vi "输入数据解析.vi"(0 "单个参数补充":dbl, 1 "从板号":dbl=1.0, 2 "主板二维码":string="BNET01", 3 "从板二维码":string="BNET01", 5 "主板引用":refnum<vi>, 7 "从板引用":refnum<vi>, 9 "主板选项":string="三级故障阀值", 11 "枚举":enum16{"主板", "从板"}(ring), 12 "快换":bool caption="快换写入") -> (4 "输出数组":dbl[][](array[numeric]), 6 "数组长度":dbl[](array[numeric]), 8 "循环次数":i32, 10 "命令":u32, 14 "名称":string[](array[string]), 15 "命令序号":u32[](array[numeric]))   [LabVIEW 2013] (continued)
                    n998 = Unbundle By Name(w2451) -> ("整组温度不均衡"=w2450:dbl)
                    n999 = call "输入分辨率计算-EV05.vi"("1字节?"=TRUE, "数值"=w2450, "偏移量"=0.0, "分辨率"=1.0) -> ("高字节1"=w2453:dbl)  [unwired: 1 in, 6 out]
                  }
                  frame Enabled {
                  }
                }
                n1000 = Build Array(w2449) -> (w2448:i32[])
              }
              frame 5 {
                # "单组电压不均衡"
                n1001 = disable-structure shown="启用" {
                  disable-tunnel: [w2465 w2468] -> w2460
                  disable-tunnel: [w2463 w2468] -> w2458
                  disable-tunnel: w2457 -> [w2462 _]
                  frame Disabled {
                    n1002 = Unbundle By Name(w2462) -> ("单组电压不均衡"=w2461:dbl)
                    n1003 = call "输入分辨率计算-EV05.vi"("1字节?"=FALSE, "数值"=w2461, "偏移量"=0.0, "分辨率"=0.001) -> ("低字节"=w2463:dbl, "高字节1"=w2465:dbl)  [unwired: 1 in, 5 out]
                  }
                  frame Enabled {
                    w2468 = 255 ("高字节1")
                  }
                }
                n1004 = Build Array(w2460, w2458) -> (w2459:i32[])
              }
              frame 6 {
                # "整组电压不均衡"
                n1005 = disable-structure shown="启用" {
                  disable-tunnel: [w2477 w2480] -> w2472
                  disable-tunnel: [w2475 w2480] -> w2470
                  disable-tunnel: w2469 -> [w2474 _]
                  frame Disabled {
                    n1006 = Unbundle By Name(w2474) -> ("整组电压不均衡"=w2473:dbl)
                    n1007 = call "输入分辨率计算-EV05.vi"("1字节?"=FALSE, "数值"=w2473, "偏移量"=0.0, "分辨率"=0.001) -> ("低字节"=w2475:dbl, "高字节1"=w2477:dbl)  [unwired: 1 in, 5 out]
                  }
                  frame Enabled {
                    w2480 = 255 ("高字节1")
                  }
                }
                n1008 = Build Array(w2472, w2470) -> (w2471:i32[])
              }
              frame 7 {
                # "单体电压过高"
                n1009 = disable-structure shown="启用" {
                  disable-tunnel: [w2489 w2492] -> w2484
                  disable-tunnel: [w2487 w2492] -> w2482
                  disable-tunnel: w2481 -> [w2486 _]
                  frame Disabled {
                    n1010 = Unbundle By Name(w2486) -> ("单体电压过高"=w2485:dbl)
                    n1011 = call "输入分辨率计算-EV05.vi"("1字节?"=FALSE, "数值"=w2485, "偏移量"=0.0, "分辨率"=0.001) -> ("低字节"=w2487:dbl, "高字节1"=w2489:dbl)  [unwired: 1 in, 5 out]
                  }
                  frame Enabled {
                    w2492 = 255 ("高字节1")
                  }
                }
                n1012 = Build Array(w2484, w2482) -> (w2483:i32[])
              }
              frame 8 {
                # "单体电压过低"
                n1013 = disable-structure shown="启用" {
                  disable-tunnel: [w2501 w2504] -> w2496
                  disable-tunnel: [w2499 w2504] -> w2494
                  disable-tunnel: w2493 -> [w2498 _]
                  frame Disabled {
                    n1014 = Unbundle By Name(w2498) -> ("单体电压过低"=w2497:dbl)
                    n1015 = call "输入分辨率计算-EV05.vi"("1字节?"=FALSE, "数值"=w2497, "偏移量"=0.0, "分辨率"=0.001) -> ("低字节"=w2499:dbl, "高字节1"=w2501:dbl)  [unwired: 1 in, 5 out]
                  }
                  frame Enabled {
                    w2504 = 255 ("高字节1")
                  }
                }
                n1016 = Build Array(w2496, w2494) -> (w2495:i32[])
              }
              frame 9 {
                # "充电电流过高"
                n1017 = disable-structure shown="启用" {
                  disable-tunnel: [w2513 w2516] -> w2508
                  disable-tunnel: [w2511 w2516] -> w2506
                  disable-tunnel: w2505 -> [w2510 _]
                  frame Disabled {
                    n1018 = Unbundle By Name(w2510) -> ("充电电流过高"=w2509:dbl)
                    n1019 = call "输入分辨率计算-EV05.vi"("1字节?"=FALSE, "数值"=w2509, "偏移量"=-3000.0, "分辨率"=0.1) -> ("低字节"=w2511:dbl, "高字节1"=w2513:dbl)  [unwired: 1 in, 5 out]
                  }
                  frame Enabled {
                    w2516 = 255 ("高字节1")
                  }
                }
                n1020 = Build Array(w2508, w2506) -> (w2507:i32[])
              }
              frame 10 {
                # "放电电流过高"
                n1021 = disable-structure shown="启用" {
                  disable-tunnel: [w2525 w2528] -> w2520
                  disable-tunnel: [w2523 w2528] -> w2518
                  disable-tunnel: w2517 -> [w2522 _]
                  frame Disabled {
                    n1022 = Unbundle By Name(w2522) -> ("放电电流过高"=w2521:dbl)
                    n1023 = call "输入分辨率计算-EV05.vi"("1字节?"=FALSE, "数值"=w2521, "偏移量"=-3000.0, "分辨率"=0.1) -> ("低字节"=w2523:dbl, "高字节1"=w2525:dbl)  [unwired: 1 in, 5 out]
                  }
                  frame Enabled {
                    w2528 = 255 ("高字节1")
                  }
                }
                n1024 = Build Array(w2520, w2518) -> (w2519:i32[])
              }
              frame 11 {
                # "单组温度不均衡"
                n1025 = disable-structure shown="启用" {
                  disable-tunnel: [w2535 255 ("高字节1")] -> w2531
                  disable-tunnel: w2529 -> [w2533 _]
                  frame Disabled {
                    n1026 = Unbundle By Name(w2533) -> ("单组温度不均衡"=w2532:dbl)
                    n1027 = call "输入分辨率计算-EV05.vi"("1字节?"=TRUE, "数值"=w2532, "偏移量"=0.0, "分辨率"=1.0) -> ("高字节1"=w2535:dbl)  [unwired: 1 in, 6 out]
                  }
                  frame Enabled {
                  }
                }
                n1028 = Build Array(w2531) -> (w2530:i32[])
              }
              frame 12 {
                # "SOC过高"
                n1029 = Unbundle By Name(w2543) -> ("SOC过高"=w2542:dbl)
                n1030 = call "输入分辨率计算-EV05.vi"("1字节?"=FALSE, "数值"=w2542, "偏移量"=0.0, "分辨率"=0.1) -> ("低字节"=w2544:dbl, "高字节1"=w2545:dbl)  [unwired: 1 in, 5 out]
                n1031 = call "二进制解析-8.6.vi"("索引"=4, "数值"=w2545) -> ("低位子数组"=w2548:i32[])  [unwired: 3 out]
                n1032 = call "二进制解析-8.6.vi"("索引"=4, "数值"=w2544) -> ("低位子数组"=w2540:i32[], "高位子数组"=w2547:i32[])  [unwired: 2 out]
                n1033 = Insert Into Array(array=w2548, new element=w2547) -> (w2546:i32[])  [unwired: 1 in]
                n1034 = call "数值二进制转十进制-8.6.vi"("子数组"=w2546) -> ("十进制数值"=w2541:i32)  [unwired: 4 out]
                n1035 = disable-structure shown="启用" {
                  disable-tunnel: w2541 -> [w2556 _]
                  disable-tunnel: [w2556 255 ("高字节1")] -> w2539
                  disable-tunnel: [w2555 i32[] [] ("低位子数组 20")] -> _
                  disable-tunnel: w2540 -> [w2555 _]
                  frame Disabled {
                  }
                  frame Enabled {
                  }
                }
                n1036 = Build Array(w2539, w2539) -> (w2552:i32[])
              }
              frame 13 {
                # "SOC过低"
                n1037 = Unbundle By Name(w2565) -> ("SOC过低"=w2564:dbl)
                n1038 = call "输入分辨率计算-EV05.vi"("1字节?"=FALSE, "数值"=w2564, "偏移量"=0.0, "分辨率"=0.1) -> ("低字节"=w2562:dbl, "高字节1"=w2563:dbl)  [unwired: 1 in, 5 out]
                n1039 = call "二进制解析-8.6.vi"("索引"=4, "数值"=w2563) -> ("低位子数组"=w2560:i32[])  [unwired: 3 out]
                n1040 = disable-structure shown="启用" {
                  disable-tunnel: w2562 -> [w2572 _]
                  disable-tunnel: [w2572 255 ("高字节1")] -> w2561
                  disable-tunnel: w2560 -> [w2571 _]
                  disable-tunnel: [_ 255 ("高字节1")] -> w2559
                  frame Disabled {
                    (unwired) i32[] [] ("低位子数组 4")
                  }
                  frame Enabled {
                  }
                }
                n1041 = Build Array(w2559, w2561) -> (w2568:i32[])
              }
              frame 14 {
                # "内阻过大"
                n1042 = disable-structure shown="启用" {
                  disable-tunnel: w2577 -> [w2582 _]
                  disable-tunnel: [w2578 255 ("高字节1")] -> w2575
                  frame Disabled {
                    n1043 = Unbundle By Name(w2582) -> ("内阻过大"=w2581:dbl)
                    n1044 = call "输入分辨率计算-EV05.vi"("1字节?"=TRUE, "数值"=w2581, "分辨率"=0.1) -> ("高字节1"=w2578:dbl)  [unwired: 2 in, 6 out]
                  }
                  frame Enabled {
                  }
                }
                n1045 = Build Array(w2575) -> (w2576:i32[])
              }
              frame 15 {
                # "极柱温度过高"
                n1046 = disable-structure shown="启用" {
                  disable-tunnel: w2586 -> [w2592 _]
                  disable-tunnel: [w2588 255 ("高字节1")] -> w2584
                  frame Disabled {
                    n1047 = Unbundle By Name(w2592) -> ("极柱温度过高"=w2591:dbl)
                    n1048 = call "输入分辨率计算-EV05.vi"("1字节?"=TRUE, "数值"=w2591, "偏移量"=-40.0, "分辨率"=1.0) -> ("高字节1"=w2588:dbl)  [unwired: 1 in, 6 out]
                  }
                  frame Enabled {
                  }
                }
                n1049 = Build Array(w2584) -> (w2585:i32[])
              }
              frame 16 {
                # "SOH过低"
                n1050 = disable-structure shown="启用" {
                  disable-tunnel: [w2609 w2617] -> w2596
                  disable-tunnel: w2595 -> [w2606 _]
                  disable-tunnel: [w2598 w2617] -> w2594
                  frame Disabled {
                    n1051 = Unbundle By Name(w2606) -> ("SOH过低"=w2605:dbl)
                    n1052 = call "输入分辨率计算-EV05.vi"("1字节?"=FALSE, "数值"=w2605, "偏移量"=0.0, "分辨率"=0.1) -> ("低字节"=w2607:dbl, "高字节1"=w2608:dbl)  [unwired: 1 in, 5 out]
                    n1053 = call "二进制解析-8.6.vi"("索引"=4, "数值"=w2608) -> ("低位子数组"=w2611:i32[])  [unwired: 3 out]
                    n1054 = call "二进制解析-8.6.vi"("索引"=4, "数值"=w2607) -> ("低位子数组"=w2600:i32[], "高位子数组"=w2610:i32[])  [unwired: 2 out]
                    n1055 = call "二进制解析-8.6.vi"("索引"=4, "数值"=0) -> ("低位子数组"=w2601:i32[])  [unwired: 3 out]
                    n1056 = Insert Into Array(array=w2611, new element=w2610) -> (w2604:i32[])  [unwired: 1 in]
                    n1057 = Insert Into Array(array=w2600, new element=w2601) -> (w2599:i32[])  [unwired: 1 in]
                    n1058 = call "数值二进制转十进制-8.6.vi"("子数组"=w2604) -> ("十进制数值"=w2609:i32)  [unwired: 4 out]
                    n1059 = call "数值二进制转十进制-8.6.vi"("子数组"=w2599) -> ("十进制数值"=w2598:i32)  [unwired: 4 out]
                  }
                  frame Enabled {
                    w2617 = 255 ("高字节1")
                  }
                }
                n1060 = Build Array(w2596, w2594) -> (w2597:i32[])
              }
            }
            n1061 = Insert Into Array(array=w2401, new element=w2402) -> (w2400:dbl[])  [unwired: 1 in]
          }
          n1062 = Build Array(w2397) -> (w2396:dbl[][])
          n1063 = Build Array("三级故障阀值") -> (w2387:string[])
        }
        frame "温度过高(2)" {
          n1064 = Unbundle By Name(w2623) -> ("一级故障 2"=w2624:refnum<vi>)
          n1065 = property class="Clust (严格)"(reference=w2624) -> ("Value"=w2622:T4)  [unwired: 1 in, 2 out]
          n1066 = for {
            N: 17 -> [_]
            tunnel: w2622 -> [w2634]
            shift-right: [w2631] -> w2628
            shift-left: dbl[] [] -> [w2632]
            i -> [w2635]
            n1067 = case shown="13" w2635 {
              tunnel: w2634 -> [w2636 w2647 w2658 w2668 w2678 w2688 w2700 w2712 w2724 w2736 w2748 w2760 w2774 w2796 w2808 w2817 w2826]
              tunnel: [w2637 w2648 w2659 w2669 w2679 w2690 w2702 w2714 w2726 w2738 w2750 w2761 w2783 w2799 w2807 w2816 w2828] -> w2633
              frame 0, Default {
                # "总电压过高"
                n1068 = disable-structure shown="启用" {
                  disable-tunnel: [w2643 w2646] -> w2639
                  disable-tunnel: [w2642 w2646] -> w2638
                  disable-tunnel: w2636 -> [w2641 _]
                  frame Disabled {
                    n1069 = Unbundle By Name(w2641) -> ("总电压过高"=w2640:dbl)
                    n1070 = call "输入分辨率计算-EV05.vi"("1字节?"=FALSE, "数值"=w2640, "分辨率"=0.1) -> ("低字节"=w2643:dbl, "高字节1"=w2642:dbl)  [unwired: 2 in, 5 out]
                  }
                  frame Enabled {
                    w2646 = 255 ("高字节1")
                  }
                }
                n1071 = Build Array(w2638, w2639) -> (w2637:i32[])
              }
              frame 1 {
                # "总电压过低"
                n1072 = disable-structure shown="启用" {
                  disable-tunnel: [w2654 w2657] -> w2650
                  disable-tunnel: [w2653 w2657] -> w2649
                  disable-tunnel: w2647 -> [w2652 _]
                  frame Disabled {
                    n1073 = Unbundle By Name(w2652) -> ("总电压过低"=w2651:dbl)
                    n1074 = call "输入分辨率计算-EV05.vi"("1字节?"=FALSE, "数值"=w2651, "分辨率"=0.1) -> ("低字节"=w2654:dbl, "高字节1"=w2653:dbl)  [unwired: 2 in, 5 out]
                  }
                  frame Enabled {
                    w2657 = 255 ("高字节1")
                  }
                }
                n1075 = Build Array(w2649, w2650) -> (w2648:i32[])
              }
              frame 2 {
                # "温度过高"
                n1076 = disable-structure shown="启用" {
                  disable-tunnel: [w2664 255 ("高字节1")] -> w2660
                  disable-tunnel: w2658 -> [w2662 _]
                  frame Enabled {
                    n1077 = Unbundle By Name(w2662) -> ("温度过高"=w2661:dbl)
                    n1078 = call "输入分辨率计算-EV05.vi"("1字节?"=TRUE, "数值"=w2661, "偏移量"=-40.0, "分辨率"=1.0) -> ("高字节1"=w2664:dbl)  [unwired: 1 in, 6 out]
                  }
                  frame Disabled {
                  }
                }
                n1079 = Build Array(w2660) -> (w2659:dbl[])
              }
              frame 3 {
                # "温度过低"
                n1080 = disable-structure shown="启用" {
                  disable-tunnel: [w2674 255 ("高字节1")] -> w2670
                  disable-tunnel: w2668 -> [w2672 _]
                  frame Disabled {
                    n1081 = Unbundle By Name(w2672) -> ("温度过低"=w2671:dbl)
                    n1082 = call "输入分辨率计算-EV05.vi"("1字节?"=TRUE, "数值"=w2671, "偏移量"=-40.0, "分辨率"=1.0) -> ("高字节1"=w2674:dbl)  [unwired: 1 in, 6 out]
                  }
                  frame Enabled {
                  }
                }
                n1083 = Build Array(w2670) -> (w2669:i32[])
              }
              frame 4 {
                # "整组温度不均衡"
                n1084 = disable-structure shown="启用" {
                  disable-tunnel: [w2684 255 ("高字节1")] -> w2680
                  disable-tunnel: w2678 -> [w2682 _]
                  frame Disabled {
                    n1085 = Unbundle By Name(w2682) -> ("整组温度不均衡"=w2681:dbl)
                    n1086 = call "输入分辨率计算-EV05.vi"("1字节?"=TRUE, "数值"=w2681, "偏移量"=0.0, "分辨率"=1.0) -> ("高字节1"=w2684:dbl)  [unwired: 1 in, 6 out]
                  }
                  frame Enabled {
                  }
                }
                n1087 = Build Array(w2680) -> (w2679:i32[])
              }
              frame 5 {
                # "单组电压不均衡"
                n1088 = disable-structure shown="启用" {
                  disable-tunnel: [w2696 w2699] -> w2691
                  disable-tunnel: [w2694 w2699] -> w2689
                  disable-tunnel: w2688 -> [w2693 _]
                  frame Disabled {
                    n1089 = Unbundle By Name(w2693) -> ("单组电压不均衡"=w2692:dbl)
                    n1090 = call "输入分辨率计算-EV05.vi"("1字节?"=FALSE, "数值"=w2692, "偏移量"=0.0, "分辨率"=0.001) -> ("低字节"=w2694:dbl, "高字节1"=w2696:dbl)  [unwired: 1 in, 5 out]
                  }
                  frame Enabled {
                    w2699 = 255 ("高字节1")
                  }
                }
                n1091 = Build Array(w2691, w2689) -> (w2690:i32[])
              }
              frame 6 {
                # "整组电压不均衡"
                n1092 = disable-structure shown="启用" {
                  disable-tunnel: [w2708 w2711] -> w2703
                  disable-tunnel: [w2706 w2711] -> w2701
                  disable-tunnel: w2700 -> [w2705 _]
                  frame Disabled {
                    n1093 = Unbundle By Name(w2705) -> ("整组电压不均衡"=w2704:dbl)
                    n1094 = call "输入分辨率计算-EV05.vi"("1字节?"=FALSE, "数值"=w2704, "偏移量"=0.0, "分辨率"=0.001) -> ("低字节"=w2706:dbl, "高字节1"=w2708:dbl)  [unwired: 1 in, 5 out]
                  }
                  frame Enabled {
                    w2711 = 255 ("高字节1")
                  }
                }
                n1095 = Build Array(w2703, w2701) -> (w2702:i32[])
              }
              frame 7 {
                # "单体电压过高"
                n1096 = disable-structure shown="启用" {
                  disable-tunnel: [w2720 w2723] -> w2715
                  disable-tunnel: [w2718 w2723] -> w2713
                  disable-tunnel: w2712 -> [w2717 _]
                  frame Disabled {
                    n1097 = Unbundle By Name(w2717) -> ("单体电压过高"=w2716:dbl)
                    n1098 = call "输入分辨率计算-EV05.vi"("1字节?"=FALSE, "数值"=w2716, "偏移量"=0.0, "分辨率"=0.001) -> ("低字节"=w2718:dbl, "高字节1"=w2720:dbl)  [unwired: 1 in, 5 out]
                  }
                  frame Enabled {
                    w2723 = 255 ("高字节1")
                  }
                }
                n1099 = Build Array(w2715, w2713) -> (w2714:i32[])
              }
              frame 8 {
                # "单体电压过低"
                n1100 = disable-structure shown="启用" {
                  disable-tunnel: [w2732 w2735] -> w2727
                  disable-tunnel: [w2730 w2735] -> w2725
                  disable-tunnel: w2724 -> [w2729 _]
                  frame Disabled {
                    n1101 = Unbundle By Name(w2729) -> ("单体电压过低"=w2728:dbl)
                    n1102 = call "输入分辨率计算-EV05.vi"("1字节?"=FALSE, "数值"=w2728, "偏移量"=0.0, "分辨率"=0.001) -> ("低字节"=w2730:dbl, "高字节1"=w2732:dbl)  [unwired: 1 in, 5 out]
                  }
                  frame Enabled {
                    w2735 = 255 ("高字节1")
                  }
                }
                n1103 = Build Array(w2727, w2725) -> (w2726:i32[])
              }
              frame 9 {
                # "充电电流过高"
                n1104 = disable-structure shown="启用" {
                  disable-tunnel: [w2744 w2747] -> w2739
                  disable-tunnel: [w2742 w2747] -> w2737
                  disable-tunnel: w2736 -> [w2741 _]
                  frame Disabled {
                    n1105 = Unbundle By Name(w2741) -> ("充电电流过高"=w2740:dbl)
                    n1106 = call "输入分辨率计算-EV05.vi"("1字节?"=FALSE, "数值"=w2740, "偏移量"=-3000.0, "分辨率"=0.1) -> ("低字节"=w2742:dbl, "高字节1"=w2744:dbl)  [unwired: 1 in, 5 out]
                  }
                  frame Enabled {
                    w2747 = 255 ("高字节1")
                  }
                }
                n1107 = Build Array(w2739, w2737) -> (w2738:i32[])
              }
              frame 10 {
                # "放电电流过高"
                n1108 = disable-structure shown="启用" {
                  disable-tunnel: [w2756 w2759] -> w2751
                  disable-tunnel: [w2754 w2759] -> w2749
                  disable-tunnel: w2748 -> [w2753 _]
                  frame Disabled {
                    n1109 = Unbundle By Name(w2753) -> ("放电电流过高"=w2752:dbl)
                    n1110 = call "输入分辨率计算-EV05.vi"("1字节?"=FALSE, "数值"=w2752, "偏移量"=-3000.0, "分辨率"=0.1) -> ("低字节"=w2754:dbl, "高字节1"=w2756:dbl)  [unwired: 1 in, 5 out]
                  }
                  frame Enabled {
                    w2759 = 255 ("高字节1")
                  }
                }
                n1111 = Build Array(w2751, w2749) -> (w2750:i32[])
              }
              frame 11 {
                # "单组温度不均衡"
                n1112 = disable-structure shown="启用" {
                  disable-tunnel: [w2766 255 ("高字节1")] -> w2762
                  disable-tunnel: w2760 -> [w2764 _]
                  frame Disabled {
                    n1113 = Unbundle By Name(w2764) -> ("单组温度不均衡"=w2763:dbl)
                    n1114 = call "输入分辨率计算-EV05.vi"("1字节?"=TRUE, "数值"=w2763, "偏移量"=0.0, "分辨率"=1.0) -> ("高字节1"=w2766:dbl)  [unwired: 1 in, 6 out]
                  }
                  frame Enabled {
                  }
                }
                n1115 = Build Array(w2762) -> (w2761:i32[])
              }
              frame 12 {
                # "SOC过高"
                n1116 = Unbundle By Name(w2774) -> ("SOC过高"=w2773:dbl)
                n1117 = call "输入分辨率计算-EV05.vi"("1字节?"=FALSE, "数值"=w2773, "偏移量"=0.0, "分辨率"=0.1) -> ("低字节"=w2775:dbl, "高字节1"=w2776:dbl)  [unwired: 1 in, 5 out]
                n1118 = call "二进制解析-8.6.vi"("索引"=4, "数值"=w2776) -> ("低位子数组"=w2779:i32[])  [unwired: 3 out]
                n1119 = call "二进制解析-8.6.vi"("索引"=4, "数值"=w2775) -> ("低位子数组"=w2771:i32[], "高位子数组"=w2778:i32[])  [unwired: 2 out]
                n1120 = Insert Into Array(array=w2779, new element=w2778) -> (w2777:i32[])  [unwired: 1 in]
                n1121 = call "数值二进制转十进制-8.6.vi"("子数组"=w2777) -> ("十进制数值"=w2772:i32)  [unwired: 4 out]
                n1122 = disable-structure shown="启用" {
                  disable-tunnel: w2772 -> [w2787 _]
                  disable-tunnel: [w2787 255 ("高字节1")] -> w2770
                  disable-tunnel: [w2786 i32[] [] ("低位子数组 20")] -> _
                  disable-tunnel: w2771 -> [w2786 _]
                  frame Disabled {
                  }
                  frame Enabled {
                  }
                }
                n1123 = Build Array(w2770, w2770) -> (w2783:i32[])
              }
              frame 13 {
                # "SOC过低"
                n1124 = Unbundle By Name(w2796) -> ("SOC过低"=w2795:dbl)
                n1125 = call "输入分辨率计算-EV05.vi"("1字节?"=FALSE, "数值"=w2795, "偏移量"=0.0, "分辨率"=0.1) -> ("低字节"=w2793:dbl, "高字节1"=w2794:dbl)  [unwired: 1 in, 5 out]
                n1126 = call "二进制解析-8.6.vi"("索引"=4, "数值"=w2794) -> ("低位子数组"=w2791:i32[])  [unwired: 3 out]
                n1127 = disable-structure shown="启用" {
                  disable-tunnel: w2793 -> [w2803 _]
                  disable-tunnel: [w2803 255 ("高字节1")] -> w2792
                  disable-tunnel: w2791 -> [w2802 _]
                  disable-tunnel: [_ 255 ("高字节1")] -> w2790
                  frame Disabled {
                    (unwired) i32[] [] ("低位子数组 4")
                  }
                  frame Enabled {
                  }
                }
                n1128 = Build Array(w2790, w2792) -> (w2799:i32[])
              }
              frame 14 {
                # "内阻过大"
                n1129 = disable-structure shown="启用" {
                  disable-tunnel: w2808 -> [w2813 _]
                  disable-tunnel: [w2809 255 ("高字节1")] -> w2806
                  frame Disabled {
                    n1130 = Unbundle By Name(w2813) -> ("内阻过大"=w2812:dbl)
                    n1131 = call "输入分辨率计算-EV05.vi"("1字节?"=TRUE, "数值"=w2812, "分辨率"=0.1) -> ("高字节1"=w2809:dbl)  [unwired: 2 in, 6 out]
                  }
                  frame Enabled {
                  }
                }
                n1132 = Build Array(w2806) -> (w2807:i32[])
              }
              frame 15 {
                # "极柱温度过高"
                n1133 = disable-structure shown="启用" {
                  disable-tunnel: w2817 -> [w2823 _]
                  disable-tunnel: [w2819 255 ("高字节1")] -> w2815
                  frame Disabled {
                    n1134 = Unbundle By Name(w2823) -> ("极柱温度过高"=w2822:dbl)
                    n1135 = call "输入分辨率计算-EV05.vi"("1字节?"=TRUE, "数值"=w2822, "偏移量"=-40.0, "分辨率"=1.0) -> ("高字节1"=w2819:dbl)  [unwired: 1 in, 6 out]
                  }
                  frame Enabled {
                  }
                }
                n1136 = Build Array(w2815) -> (w2816:i32[])
              }
              frame 16 {
                # "SOH过低"
                n1137 = disable-structure shown="启用" {
                  disable-tunnel: [w2840 w2848] -> w2827
                  disable-tunnel: w2826 -> [w2837 _]
                  disable-tunnel: [w2829 w2848] -> w2825
                  frame Disabled {
                    n1138 = Unbundle By Name(w2837) -> ("SOH过低"=w2836:dbl)
                    n1139 = call "输入分辨率计算-EV05.vi"("1字节?"=FALSE, "数值"=w2836, "偏移量"=0.0, "分辨率"=0.1) -> ("低字节"=w2838:dbl, "高字节1"=w2839:dbl)  [unwired: 1 in, 5 out]
                    n1140 = call "二进制解析-8.6.vi"("索引"=4, "数值"=w2839) -> ("低位子数组"=w2842:i32[])  [unwired: 3 out]
                    n1141 = call "二进制解析-8.6.vi"("索引"=4, "数值"=w2838) -> ("低位子数组"=w2831:i32[], "高位子数组"=w2841:i32[])  [unwired: 2 out]
                    n1142 = call "二进制解析-8.6.vi"("索引"=4, "数值"=0) -> ("低位子数组"=w2832:i32[])  [unwired: 3 out]
                    n1143 = Insert Into Array(array=w2842, new element=w2841) -> (w2835:i32[])  [unwired: 1 in]
                    n1144 = Insert Into Array(array=w2831, new element=w2832) -> (w2830:i32[])  [unwired: 1 in]
                    n1145 = call "数值二进制转十进制-8.6.vi"("子数组"=w2835) -> ("十进制数值"=w2840:i32)  [unwired: 4 out]
                    n1146 = call "数值二进制转十进制-8.6.vi"("子数组"=w2830) -> ("十进制数值"=w2829:i32)  [unwired: 4 out]
                  }
                  frame Enabled {
                    w2848 = 255 ("高字节1")
                  }
                }
                n1147 = Build Array(w2827, w2825) -> (w2828:i32[])
              }
            }
            n1148 = Insert Into Array(array=w2632, new element=w2633) -> (w2631:dbl[])  [unwired: 1 in]
          }
          n1149 = Build Array(w2628) -> (w2627:dbl[][])
          n1150 = Build Array("二级故障阀值") -> (w2618:string[])
        }
        frame "温度过高(3)" {
          n1151 = Unbundle By Name(w2854) -> ("一级故障 3"=w2855:refnum<vi>)
          n1152 = property class="Clust (严格)"(reference=w2855) -> ("Value"=w2853:T4)  [unwired: 1 in, 2 out]
          n1153 = for {
            N: 17 -> [_]
            tunnel: w2853 -> [w2865]
            shift-right: [w2862] -> w2859
            shift-left: dbl[] [] -> [w2863]
            i -> [w2866]
            n1154 = case shown="13" w2866 {
              tunnel: w2865 -> [w2867 w2878 w2889 w2899 w2909 w2919 w2931 w2943 w2955 w2967 w2979 w2991 w3005 w3027 w3039 w3048 w3057]
              tunnel: [w2868 w2879 w2890 w2900 w2910 w2921 w2933 w2945 w2957 w2969 w2981 w2992 w3014 w3030 w3038 w3047 w3059] -> w2864
              frame 0, Default {
                # "总电压过高"
                n1155 = disable-structure shown="启用" {
                  disable-tunnel: [w2874 w2877] -> w2870
                  disable-tunnel: [w2873 w2877] -> w2869
                  disable-tunnel: w2867 -> [w2872 _]
                  frame Disabled {
                    n1156 = Unbundle By Name(w2872) -> ("总电压过高"=w2871:dbl)
                    n1157 = call "输入分辨率计算-EV05.vi"("1字节?"=FALSE, "数值"=w2871, "分辨率"=0.1) -> ("低字节"=w2874:dbl, "高字节1"=w2873:dbl)  [unwired: 2 in, 5 out]
                  }
                  frame Enabled {
                    w2877 = 255 ("高字节1")
                  }
                }
                n1158 = Build Array(w2869, w2870) -> (w2868:i32[])
              }
              frame 1 {
                # "总电压过低"
                n1159 = disable-structure shown="启用" {
                  disable-tunnel: [w2885 w2888] -> w2881
                  disable-tunnel: [w2884 w2888] -> w2880
                  disable-tunnel: w2878 -> [w2883 _]
                  frame Disabled {
                    n1160 = Unbundle By Name(w2883) -> ("总电压过低"=w2882:dbl)
                    n1161 = call "输入分辨率计算-EV05.vi"("1字节?"=FALSE, "数值"=w2882, "分辨率"=0.1) -> ("低字节"=w2885:dbl, "高字节1"=w2884:dbl)  [unwired: 2 in, 5 out]
                  }
                  frame Enabled {
                    w2888 = 255 ("高字节1")
                  }
                }
                n1162 = Build Array(w2880, w2881) -> (w2879:i32[])
              }
              frame 2 {
                # "温度过高"
                n1163 = disable-structure shown="启用" {
                  disable-tunnel: [w2895 255 ("高字节1")] -> w2891
                  disable-tunnel: w2889 -> [w2893 _]
                  frame Enabled {
                    n1164 = Unbundle By Name(w2893) -> ("温度过高"=w2892:dbl)
                    n1165 = call "输入分辨率计算-EV05.vi"("1字节?"=TRUE, "数值"=w2892, "偏移量"=-40.0, "分辨率"=1.0) -> ("高字节1"=w2895:dbl)  [unwired: 1 in, 6 out]
                  }
                  frame Disabled {
                  }
                }
                n1166 = Build Array(w2891) -> (w2890:dbl[])
              }
              frame 3 {
                # "温度过低"
                n1167 = disable-structure shown="启用" {
                  disable-tunnel: [w2905 255 ("高字节1")] -> w2901
                  disable-tunnel: w2899 -> [w2903 _]
                  frame Disabled {
                    n1168 = Unbundle By Name(w2903) -> ("温度过低"=w2902:dbl)
                    n1169 = call "输入分辨率计算-EV05.vi"("1字节?"=TRUE, "数值"=w2902, "偏移量"=-40.0, "分辨率"=1.0) -> ("高字节1"=w2905:dbl)  [unwired: 1 in, 6 out]
                  }
                  frame Enabled {
                  }
                }
                n1170 = Build Array(w2901) -> (w2900:i32[])
              }
              frame 4 {
                # "整组温度不均衡"
                n1171 = disable-structure shown="启用" {
                  disable-tunnel: [w2915 255 ("高字节1")] -> w2911
                  disable-tunnel: w2909 -> [w2913 _]
                  frame Disabled {
                    n1172 = Unbundle By Name(w2913) -> ("整组温度不均衡"=w2912:dbl)
                    n1173 = call "输入分辨率计算-EV05.vi"("1字节?"=TRUE, "数值"=w2912, "偏移量"=0.0, "分辨率"=1.0) -> ("高字节1"=w2915:dbl)  [unwired: 1 in, 6 out]
                  }
                  frame Enabled {
                  }
                }
                n1174 = Build Array(w2911) -> (w2910:i32[])
              }
              frame 5 {
                # "单组电压不均衡"
                n1175 = disable-structure shown="启用" {
                  disable-tunnel: [w2927 w2930] -> w2922
                  disable-tunnel: [w2925 w2930] -> w2920
                  disable-tunnel: w2919 -> [w2924 _]
                  frame Disabled {
                    n1176 = Unbundle By Name(w2924) -> ("单组电压不均衡"=w2923:dbl)
                    n1177 = call "输入分辨率计算-EV05.vi"("1字节?"=FALSE, "数值"=w2923, "偏移量"=0.0, "分辨率"=0.001) -> ("低字节"=w2925:dbl, "高字节1"=w2927:dbl)  [unwired: 1 in, 5 out]
                  }
                  frame Enabled {
                    w2930 = 255 ("高字节1")
                  }
                }
                n1178 = Build Array(w2922, w2920) -> (w2921:i32[])
              }
              frame 6 {
                # "整组电压不均衡"
                n1179 = disable-structure shown="启用" {
                  disable-tunnel: [w2939 w2942] -> w2934
                  disable-tunnel: [w2937 w2942] -> w2932
                  disable-tunnel: w2931 -> [w2936 _]
                  frame Disabled {
                    n1180 = Unbundle By Name(w2936) -> ("整组电压不均衡"=w2935:dbl)
                    n1181 = call "输入分辨率计算-EV05.vi"("1字节?"=FALSE, "数值"=w2935, "偏移量"=0.0, "分辨率"=0.001) -> ("低字节"=w2937:dbl, "高字节1"=w2939:dbl)  [unwired: 1 in, 5 out]
                  }
                  frame Enabled {
                    w2942 = 255 ("高字节1")
                  }
                }
                n1182 = Build Array(w2934, w2932) -> (w2933:i32[])
              }
              frame 7 {
                # "单体电压过高"
                n1183 = disable-structure shown="启用" {
                  disable-tunnel: [w2951 w2954] -> w2946
                  disable-tunnel: [w2949 w2954] -> w2944
                  disable-tunnel: w2943 -> [w2948 _]
                  frame Disabled {
                    n1184 = Unbundle By Name(w2948) -> ("单体电压过高"=w2947:dbl)
                    n1185 = call "输入分辨率计算-EV05.vi"("1字节?"=FALSE, "数值"=w2947, "偏移量"=0.0, "分辨率"=0.001) -> ("低字节"=w2949:dbl, "高字节1"=w2951:dbl)  [unwired: 1 in, 5 out]
                  }
                  frame Enabled {
                    w2954 = 255 ("高字节1")
                  }
                }
                n1186 = Build Array(w2946, w2944) -> (w2945:i32[])
              }
              frame 8 {
                # "单体电压过低"
                n1187 = disable-structure shown="启用" {
                  disable-tunnel: [w2963 w2966] -> w2958
                  disable-tunnel: [w2961 w2966] -> w2956
                  disable-tunnel: w2955 -> [w2960 _]
                  frame Disabled {
                    n1188 = Unbundle By Name(w2960) -> ("单体电压过低"=w2959:dbl)
                    n1189 = call "输入分辨率计算-EV05.vi"("1字节?"=FALSE, "数值"=w2959, "偏移量"=0.0, "分辨率"=0.001) -> ("低字节"=w2961:dbl, "高字节1"=w2963:dbl)  [unwired: 1 in, 5 out]
                  }
                  frame Enabled {
                    w2966 = 255 ("高字节1")
                  }
                }
                n1190 = Build Array(w2958, w2956) -> (w2957:i32[])
              }
              frame 9 {
                # "充电电流过高"
                n1191 = disable-structure shown="启用" {
                  disable-tunnel: [w2975 w2978] -> w2970
                  disable-tunnel: [w2973 w2978] -> w2968
                  disable-tunnel: w2967 -> [w2972 _]
                  frame Disabled {
                    n1192 = Unbundle By Name(w2972) -> ("充电电流过高"=w2971:dbl)
                    n1193 = call "输入分辨率计算-EV05.vi"("1字节?"=FALSE, "数值"=w2971, "偏移量"=-3000.0, "分辨率"=0.1) -> ("低字节"=w2973:dbl, "高字节1"=w2975:dbl)  [unwired: 1 in, 5 out]
                  }
                  frame Enabled {
                    w2978 = 255 ("高字节1")
                  }
                }
                n1194 = Build Array(w2970, w2968) -> (w2969:i32[])
              }
              frame 10 {
                # "放电电流过高"
                n1195 = disable-structure shown="启用" {
                  disable-tunnel: [w2987 w2990] -> w2982
                  disable-tunnel: [w2985 w2990] -> w2980
                  disable-tunnel: w2979 -> [w2984 _]
                  frame Disabled {
                    n1196 = Unbundle By Name(w2984) -> ("放电电流过高"=w2983:dbl)
                    n1197 = call "输入分辨率计算-EV05.vi"("1字节?"=FALSE, "数值"=w2983, "偏移量"=-3000.0, "分辨率"=0.1) -> ("低字节"=w2985:dbl, "高字节1"=w2987:dbl)  [unwired: 1 in, 5 out]
                  }
                  frame Enabled {
                    w2990 = 255 ("高字节1")
                  }
                }
                n1198 = Build Array(w2982, w2980) -> (w2981:i32[])
              }
              frame 11 {
                # "单组温度不均衡"
                n1199 = disable-structure shown="启用" {
                  disable-tunnel: [w2997 255 ("高字节1")] -> w2993
                  disable-tunnel: w2991 -> [w2995 _]
                  frame Disabled {
                    n1200 = Unbundle By Name(w2995) -> ("单组温度不均衡"=w2994:dbl)
                    n1201 = call "输入分辨率计算-EV05.vi"("1字节?"=TRUE, "数值"=w2994, "偏移量"=0.0, "分辨率"=1.0) -> ("高字节1"=w2997:dbl)  [unwired: 1 in, 6 out]
                  }
                  frame Enabled {
                  }
                }
                n1202 = Build Array(w2993) -> (w2992:i32[])
              }
              frame 12 {
                # "SOC过高"
                n1203 = Unbundle By Name(w3005) -> ("SOC过高"=w3004:dbl)
                n1204 = call "输入分辨率计算-EV05.vi"("1字节?"=FALSE, "数值"=w3004, "偏移量"=0.0, "分辨率"=0.1) -> ("低字节"=w3006:dbl, "高字节1"=w3007:dbl)  [unwired: 1 in, 5 out]
                n1205 = call "二进制解析-8.6.vi"("索引"=4, "数值"=w3007) -> ("低位子数组"=w3010:i32[])  [unwired: 3 out]
                n1206 = call "二进制解析-8.6.vi"("索引"=4, "数值"=w3006) -> ("低位子数组"=w3002:i32[], "高位子数组"=w3009:i32[])  [unwired: 2 out]
                n1207 = Insert Into Array(array=w3010, new element=w3009) -> (w3008:i32[])  [unwired: 1 in]
                n1208 = call "数值二进制转十进制-8.6.vi"("子数组"=w3008) -> ("十进制数值"=w3003:i32)  [unwired: 4 out]
                n1209 = disable-structure shown="启用" {
                  disable-tunnel: w3003 -> [w3018 _]
                  disable-tunnel: [w3018 255 ("高字节1")] -> w3001
                  disable-tunnel: [w3017 i32[] [] ("低位子数组 20")] -> _
                  disable-tunnel: w3002 -> [w3017 _]
                  frame Disabled {
                  }
                  frame Enabled {
                  }
                }
                n1210 = Build Array(w3001, w3001) -> (w3014:i32[])
              }
              frame 13 {
                # "SOC过低"
                n1211 = Unbundle By Name(w3027) -> ("SOC过低"=w3026:dbl)
                n1212 = call "输入分辨率计算-EV05.vi"("1字节?"=FALSE, "数值"=w3026, "偏移量"=0.0, "分辨率"=0.1) -> ("低字节"=w3024:dbl, "高字节1"=w3025:dbl)  [unwired: 1 in, 5 out]
                n1213 = call "二进制解析-8.6.vi"("索引"=4, "数值"=w3025) -> ("低位子数组"=w3022:i32[])  [unwired: 3 out]
                n1214 = disable-structure shown="启用" {
                  disable-tunnel: w3024 -> [w3034 _]
                  disable-tunnel: [w3034 255 ("高字节1")] -> w3023
                  disable-tunnel: w3022 -> [w3033 _]
                  disable-tunnel: [_ 255 ("高字节1")] -> w3021
                  frame Disabled {
                    (unwired) i32[] [] ("低位子数组 4")
                  }
                  frame Enabled {
                  }
                }
                n1215 = Build Array(w3021, w3023) -> (w3030:i32[])
              }
              frame 14 {
                # "内阻过大"
                n1216 = disable-structure shown="启用" {
                  disable-tunnel: w3039 -> [w3044 _]
                  disable-tunnel: [w3040 255 ("高字节1")] -> w3037
                  frame Disabled {
                    n1217 = Unbundle By Name(w3044) -> ("内阻过大"=w3043:dbl)
                    n1218 = call "输入分辨率计算-EV05.vi"("1字节?"=TRUE, "数值"=w3043, "分辨率"=0.1) -> ("高字节1"=w3040:dbl)  [unwired: 2 in, 6 out]
                  }
                  frame Enabled {
                  }
                }
                n1219 = Build Array(w3037) -> (w3038:i32[])
              }
              frame 15 {
                # "极柱温度过高"
                n1220 = disable-structure shown="启用" {
                  disable-tunnel: w3048 -> [w3054 _]
                  disable-tunnel: [w3050 255 ("高字节1")] -> w3046
                  frame Disabled {
                    n1221 = Unbundle By Name(w3054) -> ("极柱温度过高"=w3053:dbl)
                    n1222 = call "输入分辨率计算-EV05.vi"("1字节?"=TRUE, "数值"=w3053, "偏移量"=-40.0, "分辨率"=1.0) -> ("高字节1"=w3050:dbl)  [unwired: 1 in, 6 out]
                  }
                  frame Enabled {
                  }
                }
                n1223 = Build Array(w3046) -> (w3047:i32[])
              }
              frame 16 {
                # "SOH过低"
                n1224 = disable-structure shown="启用" {
                  disable-tunnel: [w3071 w3079] -> w3058
                  disable-tunnel: w3057 -> [w3068 _]
                  disable-tunnel: [w3060 w3079] -> w3056
                  frame Disabled {
                    n1225 = Unbundle By Name(w3068) -> ("SOH过低"=w3067:dbl)
                    n1226 = call "输入分辨率计算-EV05.vi"("1字节?"=FALSE, "数值"=w3067, "偏移量"=0.0, "分辨率"=0.1) -> ("低字节"=w3069:dbl, "高字节1"=w3070:dbl)  [unwired: 1 in, 5 out]
                    n1227 = call "二进制解析-8.6.vi"("索引"=4, "数值"=w3070) -> ("低位子数组"=w3073:i32[])  [unwired: 3 out]
                    n1228 = call "二进制解析-8.6.vi"("索引"=4, "数值"=w3069) -> ("低位子数组"=w3062:i32[], "高位子数组"=w3072:i32[])  [unwired: 2 out]
                    n1229 = call "二进制解析-8.6.vi"("索引"=4, "数值"=0) -> ("低位子数组"=w3063:i32[])  [unwired: 3 out]
                    n1230 = Insert Into Array(array=w3073, new element=w3072) -> (w3066:i32[])  [unwired: 1 in]
                    n1231 = Insert Into Array(array=w3062, new element=w3063) -> (w3061:i32[])  [unwired: 1 in]
                    n1232 = call "数值二进制转十进制-8.6.vi"("子数组"=w3066) -> ("十进制数值"=w3071:i32)  [unwired: 4 out]
                    n1233 = call "数值二进制转十进制-8.6.vi"("子数组"=w3061) -> ("十进制数值"=w3060:i32)  [unwired: 4 out]
                  }
                  frame Enabled {
                    w3079 = 255 ("高字节1")
                  }
                }
                n1234 = Build Array(w3058, w3056) -> (w3059:i32[])
              }
            }
            n1235 = Insert Into Array(array=w2863, new element=w2864) -> (w2862:dbl[])  [unwired: 1 in]
          }
          n1236 = Build Array(w2859) -> (w2858:dbl[][])
          n1237 = Build Array("三级故障阀值") -> (w2849:string[])
        }
        frame "温度过低" {
          n1238 = Unbundle By Name(w3085) -> ("一级故障"=w3086:refnum<vi>)
          n1239 = property class="Clust (严格)"(reference=w3086) -> ("Value"=w3084:T4)  [unwired: 1 in, 2 out]
          n1240 = for {
            N: 17 -> [_]
            tunnel: w3084 -> [w3096]
            shift-right: [w3093] -> w3090
            shift-left: dbl[] [] -> [w3094]
            i -> [w3097]
            n1241 = case shown="13" w3097 {
              tunnel: w3096 -> [w3098 w3109 w3120 w3130 w3140 w3150 w3162 w3174 w3186 w3198 w3210 w3222 w3236 w3258 w3270 w3279 w3288]
              tunnel: [w3099 w3110 w3121 w3131 w3141 w3152 w3164 w3176 w3188 w3200 w3212 w3223 w3245 w3261 w3269 w3278 w3290] -> w3095
              frame 0, Default {
                # "总电压过高"
                n1242 = disable-structure shown="启用" {
                  disable-tunnel: [w3105 w3108] -> w3101
                  disable-tunnel: [w3104 w3108] -> w3100
                  disable-tunnel: w3098 -> [w3103 _]
                  frame Disabled {
                    n1243 = Unbundle By Name(w3103) -> ("总电压过高"=w3102:dbl)
                    n1244 = call "输入分辨率计算-EV05.vi"("1字节?"=FALSE, "数值"=w3102, "分辨率"=0.1) -> ("低字节"=w3105:dbl, "高字节1"=w3104:dbl)  [unwired: 2 in, 5 out]
                  }
                  frame Enabled {
                    w3108 = 255 ("高字节1")
                  }
                }
                n1245 = Build Array(w3100, w3101) -> (w3099:i32[])
              }
              frame 1 {
                # "总电压过低"
                n1246 = disable-structure shown="启用" {
                  disable-tunnel: [w3116 w3119] -> w3112
                  disable-tunnel: [w3115 w3119] -> w3111
                  disable-tunnel: w3109 -> [w3114 _]
                  frame Disabled {
                    n1247 = Unbundle By Name(w3114) -> ("总电压过低"=w3113:dbl)
                    n1248 = call "输入分辨率计算-EV05.vi"("1字节?"=FALSE, "数值"=w3113, "分辨率"=0.1) -> ("低字节"=w3116:dbl, "高字节1"=w3115:dbl)  [unwired: 2 in, 5 out]
                  }
                  frame Enabled {
                    w3119 = 255 ("高字节1")
                  }
                }
                n1249 = Build Array(w3111, w3112) -> (w3110:i32[])
              }
              frame 2 {
                # "温度过高"
                n1250 = disable-structure shown="启用" {
                  disable-tunnel: [w3126 255 ("高字节1")] -> w3122
                  disable-tunnel: w3120 -> [w3124 _]
                  frame Disabled {
                    n1251 = Unbundle By Name(w3124) -> ("温度过高"=w3123:dbl)
                    n1252 = call "输入分辨率计算-EV05.vi"("1字节?"=TRUE, "数值"=w3123, "偏移量"=-40.0, "分辨率"=1.0) -> ("高字节1"=w3126:dbl)  [unwired: 1 in, 6 out]
                  }
                  frame Enabled {
                  }
                }
                n1253 = Build Array(w3122) -> (w3121:i32[])
              }
              frame 3 {
                # "温度过低"
                n1254 = disable-structure shown="启用" {
                  disable-tunnel: [w3136 255 ("高字节1")] -> w3132
                  disable-tunnel: w3130 -> [w3134 _]
                  frame Enabled {
                    n1255 = Unbundle By Name(w3134) -> ("温度过低"=w3133:dbl)
                    n1256 = call "输入分辨率计算-EV05.vi"("1字节?"=TRUE, "数值"=w3133, "偏移量"=-40.0, "分辨率"=1.0) -> ("高字节1"=w3136:dbl)  [unwired: 1 in, 6 out]
                  }
                  frame Disabled {
                  }
                }
                n1257 = Build Array(w3132) -> (w3131:dbl[])
              }
              frame 4 {
                # "整组温度不均衡"
                n1258 = disable-structure shown="启用" {
                  disable-tunnel: [w3146 255 ("高字节1")] -> w3142
                  disable-tunnel: w3140 -> [w3144 _]
                  frame Disabled {
                    n1259 = Unbundle By Name(w3144) -> ("整组温度不均衡"=w3143:dbl)
                    n1260 = call "输入分辨率计算-EV05.vi"("1字节?"=TRUE, "数值"=w3143, "偏移量"=0.0, "分辨率"=1.0) -> ("高字节1"=w3146:dbl)  [unwired: 1 in, 6 out]
                  }
                  frame Enabled {
                  }
                }
                n1261 = Build Array(w3142) -> (w3141:i32[])
              }
              frame 5 {
                # "单组电压不均衡"
                n1262 = disable-structure shown="启用" {
                  disable-tunnel: [w3158 w3161] -> w3153
                  disable-tunnel: [w3156 w3161] -> w3151
                  disable-tunnel: w3150 -> [w3155 _]
                  frame Disabled {
                    n1263 = Unbundle By Name(w3155) -> ("单组电压不均衡"=w3154:dbl)
                    n1264 = call "输入分辨率计算-EV05.vi"("1字节?"=FALSE, "数值"=w3154, "偏移量"=0.0, "分辨率"=0.001) -> ("低字节"=w3156:dbl, "高字节1"=w3158:dbl)  [unwired: 1 in, 5 out]
                  }
                  frame Enabled {
                    w3161 = 255 ("高字节1")
                  }
                }
                n1265 = Build Array(w3153, w3151) -> (w3152:i32[])
              }
              frame 6 {
                # "整组电压不均衡"
                n1266 = disable-structure shown="启用" {
                  disable-tunnel: [w3170 w3173] -> w3165
                  disable-tunnel: [w3168 w3173] -> w3163
                  disable-tunnel: w3162 -> [w3167 _]
                  frame Disabled {
                    n1267 = Unbundle By Name(w3167) -> ("整组电压不均衡"=w3166:dbl)
                    n1268 = call "输入分辨率计算-EV05.vi"("1字节?"=FALSE, "数值"=w3166, "偏移量"=0.0, "分辨率"=0.001) -> ("低字节"=w3168:dbl, "高字节1"=w3170:dbl)  [unwired: 1 in, 5 out]
                  }
                  frame Enabled {
                    w3173 = 255 ("高字节1")
                  }
                }
                n1269 = Build Array(w3165, w3163) -> (w3164:i32[])
              }
              frame 7 {
                # "单体电压过高"
                n1270 = disable-structure shown="启用" {
                  disable-tunnel: [w3182 w3185] -> w3177
                  disable-tunnel: [w3180 w3185] -> w3175
                  disable-tunnel: w3174 -> [w3179 _]
                  frame Disabled {
                    n1271 = Unbundle By Name(w3179) -> ("单体电压过高"=w3178:dbl)
                    n1272 = call "输入分辨率计算-EV05.vi"("1字节?"=FALSE, "数值"=w3178, "偏移量"=0.0, "分辨率"=0.001) -> ("低字节"=w3180:dbl, "高字节1"=w3182:dbl)  [unwired: 1 in, 5 out]
                  }
                  frame Enabled {
                    w3185 = 255 ("高字节1")
                  }
                }
                n1273 = Build Array(w3177, w3175) -> (w3176:i32[])
              }
              frame 8 {
                # "单体电压过低"
                n1274 = disable-structure shown="启用" {
                  disable-tunnel: [w3194 w3197] -> w3189
                  disable-tunnel: [w3192 w3197] -> w3187
                  disable-tunnel: w3186 -> [w3191 _]
                  frame Disabled {
                    n1275 = Unbundle By Name(w3191) -> ("单体电压过低"=w3190:dbl)
                    n1276 = call "输入分辨率计算-EV05.vi"("1字节?"=FALSE, "数值"=w3190, "偏移量"=0.0, "分辨率"=0.001) -> ("低字节"=w3192:dbl, "高字节1"=w3194:dbl)  [unwired: 1 in, 5 out]
                  }
                  frame Enabled {
                    w3197 = 255 ("高字节1")
                  }
                }
                n1277 = Build Array(w3189, w3187) -> (w3188:i32[])
              }
              frame 9 {
                # "充电电流过高"
                n1278 = disable-structure shown="启用" {
                  disable-tunnel: [w3206 w3209] -> w3201
                  disable-tunnel: [w3204 w3209] -> w3199
                  disable-tunnel: w3198 -> [w3203 _]
                  frame Disabled {
                    n1279 = Unbundle By Name(w3203) -> ("充电电流过高"=w3202:dbl)
                    n1280 = call "输入分辨率计算-EV05.vi"("1字节?"=FALSE, "数值"=w3202, "偏移量"=-3000.0, "分辨率"=0.1) -> ("低字节"=w3204:dbl, "高字节1"=w3206:dbl)  [unwired: 1 in, 5 out]
                  }
                  frame Enabled {
                    w3209 = 255 ("高字节1")
                  }
                }
                n1281 = Build Array(w3201, w3199) -> (w3200:i32[])
              }
              frame 10 {
                # "放电电流过高"
                n1282 = disable-structure shown="启用" {
                  disable-tunnel: [w3218 w3221] -> w3213
                  disable-tunnel: [w3216 w3221] -> w3211
                  disable-tunnel: w3210 -> [w3215 _]
                  frame Disabled {
                    n1283 = Unbundle By Name(w3215) -> ("放电电流过高"=w3214:dbl)
                    n1284 = call "输入分辨率计算-EV05.vi"("1字节?"=FALSE, "数值"=w3214, "偏移量"=-3000.0, "分辨率"=0.1) -> ("低字节"=w3216:dbl, "高字节1"=w3218:dbl)  [unwired: 1 in, 5 out]
                  }
                  frame Enabled {
                    w3221 = 255 ("高字节1")
                  }
                }
                n1285 = Build Array(w3213, w3211) -> (w3212:i32[])
              }
              frame 11 {
                # "单组温度不均衡"
                n1286 = disable-structure shown="启用" {
                  disable-tunnel: [w3228 255 ("高字节1")] -> w3224
                  disable-tunnel: w3222 -> [w3226 _]
                  frame Disabled {
                    n1287 = Unbundle By Name(w3226) -> ("单组温度不均衡"=w3225:dbl)
                    n1288 = call "输入分辨率计算-EV05.vi"("1字节?"=TRUE, "数值"=w3225, "偏移量"=0.0, "分辨率"=1.0) -> ("高字节1"=w3228:dbl)  [unwired: 1 in, 6 out]
                  }
                  frame Enabled {
                  }
                }
                n1289 = Build Array(w3224) -> (w3223:i32[])
              }
              frame 12 {
                # "SOC过高"
                n1290 = Unbundle By Name(w3236) -> ("SOC过高"=w3235:dbl)
                n1291 = call "输入分辨率计算-EV05.vi"("1字节?"=FALSE, "数值"=w3235, "偏移量"=0.0, "分辨率"=0.1) -> ("低字节"=w3237:dbl, "高字节1"=w3238:dbl)  [unwired: 1 in, 5 out]
                n1292 = call "二进制解析-8.6.vi"("索引"=4, "数值"=w3238) -> ("低位子数组"=w3241:i32[])  [unwired: 3 out]
                n1293 = call "二进制解析-8.6.vi"("索引"=4, "数值"=w3237) -> ("低位子数组"=w3233:i32[], "高位子数组"=w3240:i32[])  [unwired: 2 out]
                n1294 = Insert Into Array(array=w3241, new element=w3240) -> (w3239:i32[])  [unwired: 1 in]
                n1295 = call "数值二进制转十进制-8.6.vi"("子数组"=w3239) -> ("十进制数值"=w3234:i32)  [unwired: 4 out]
                n1296 = disable-structure shown="启用" {
                  disable-tunnel: w3234 -> [w3249 _]
                  disable-tunnel: [w3249 255 ("高字节1")] -> w3232
                  disable-tunnel: [w3248 i32[] [] ("低位子数组 21")] -> _
                  disable-tunnel: w3233 -> [w3248 _]
                  frame Disabled {
                  }
                  frame Enabled {
                  }
                }
                n1297 = Build Array(w3232, w3232) -> (w3245:i32[])
              }
              frame 13 {
                # "SOC过低"
                n1298 = Unbundle By Name(w3258) -> ("SOC过低"=w3257:dbl)
                n1299 = call "输入分辨率计算-EV05.vi"("1字节?"=FALSE, "数值"=w3257, "偏移量"=0.0, "分辨率"=0.1) -> ("低字节"=w3255:dbl, "高字节1"=w3256:dbl)  [unwired: 1 in, 5 out]
                n1300 = call "二进制解析-8.6.vi"("索引"=4, "数值"=w3256) -> ("低位子数组"=w3253:i32[])  [unwired: 3 out]
                n1301 = disable-structure shown="启用" {
                  disable-tunnel: w3255 -> [w3265 _]
                  disable-tunnel: [w3265 255 ("高字节1")] -> w3254
                  disable-tunnel: w3253 -> [w3264 _]
                  disable-tunnel: [_ 255 ("高字节1")] -> w3252
                  frame Disabled {
                    (unwired) i32[] [] ("低位子数组 4")
                  }
                  frame Enabled {
                  }
                }
                n1302 = Build Array(w3252, w3254) -> (w3261:i32[])
              }
              frame 14 {
                # "内阻过大"
                n1303 = disable-structure shown="启用" {
                  disable-tunnel: w3270 -> [w3275 _]
                  disable-tunnel: [w3271 255 ("高字节1")] -> w3268
                  frame Disabled {
                    n1304 = Unbundle By Name(w3275) -> ("内阻过大"=w3274:dbl)
                    n1305 = call "输入分辨率计算-EV05.vi"("1字节?"=TRUE, "数值"=w3274, "分辨率"=0.1) -> ("高字节1"=w3271:dbl)  [unwired: 2 in, 6 out]
                  }
                  frame Enabled {
                  }
                }
                n1306 = Build Array(w3268) -> (w3269:i32[])
              }
              frame 15 {
                # "极柱温度过高"
                n1307 = disable-structure shown="启用" {
                  disable-tunnel: w3279 -> [w3285 _]
                  disable-tunnel: [w3281 255 ("高字节1")] -> w3277
                  frame Disabled {
                    n1308 = Unbundle By Name(w3285) -> ("极柱温度过高"=w3284:dbl)
                    n1309 = call "输入分辨率计算-EV05.vi"("1字节?"=TRUE, "数值"=w3284, "偏移量"=-40.0, "分辨率"=1.0) -> ("高字节1"=w3281:dbl)  [unwired: 1 in, 6 out]
                  }
                  frame Enabled {
                  }
                }
